vi "Initialise.vi"(8 "error in (no error)":errorcluster, 9 "Distance":dbl, 10 "Speed":dbl) -> (0 "error out":errorcluster, 3 "MovementInstruction.lvclass":refnum<class "MovementInstruction.lvclass">)   [LabVIEW 2015, in "MovementInstruction.lvclass"]
uses:
  MovementInstruction.lvclass
  MovementInstruction.lvclass/MovementInstruction.ctl
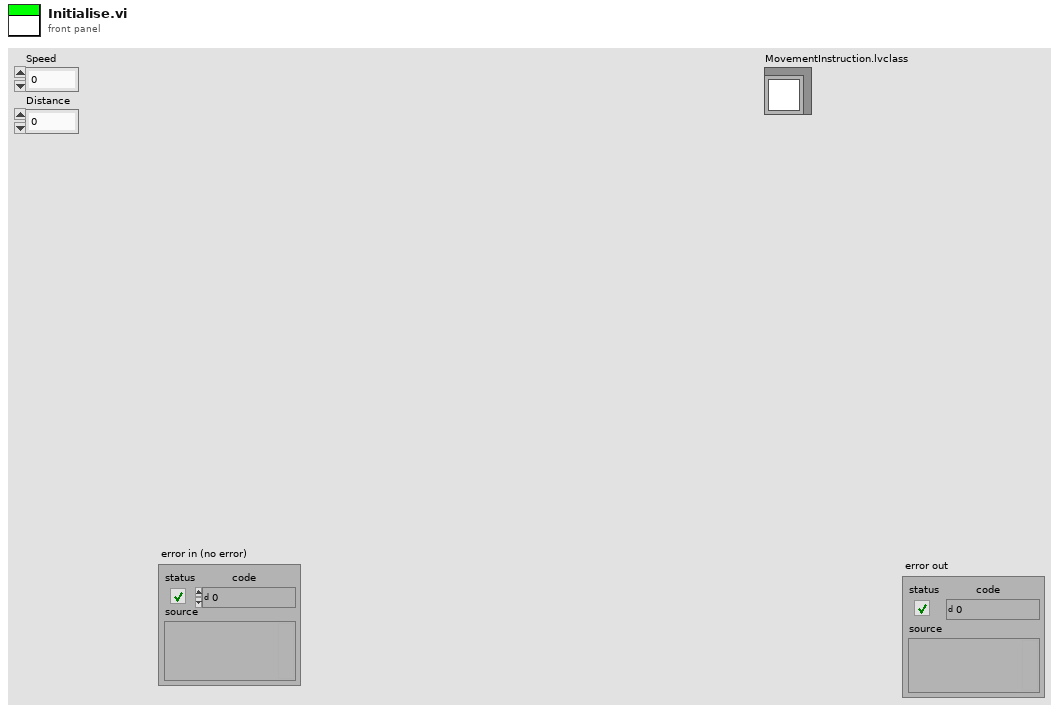
[diagram p1: front panel]
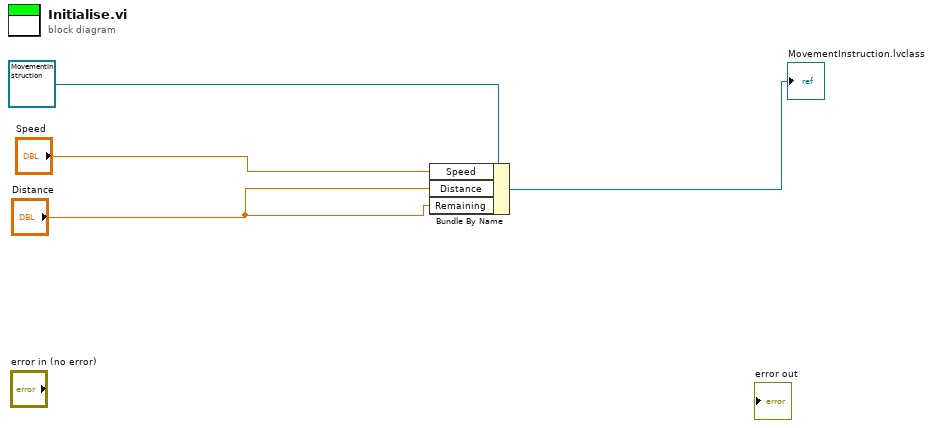
[diagram p0: block diagram]
diagram:
  n1 = Bundle By Name(cluster=refnum<class "MovementInstruction.lvclass"> refnum ("MovementInstruction.lvclass"), "Speed"="Speed", "Distance"="Distance", "Remaining"="Distance") -> (→"MovementInstruction.lvclass":refnum<class "MovementInstruction.lvclass">)
